vi "N-D TimeStamped Logging (SubVI) v1.0.vi"(8 "error in (no error)":errorcluster, 10 "array":dbl[](array[numeric]), 11 "path":path) -> (0 "error out":errorcluster)   [LabVIEW 2017]
uses:
  <vilib>/Utility/file.llb/Write Delimited Spreadsheet (string).vi
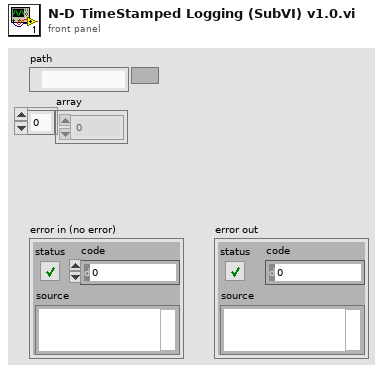
[diagram p1: front panel]
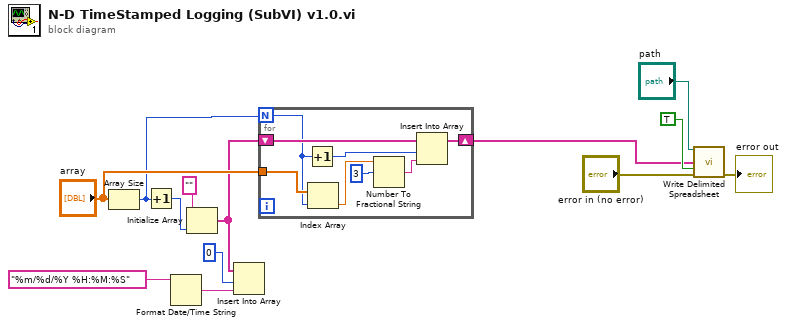
[diagram p0: block diagram]
diagram:
  n1 = Array Size(array="array") -> (size(s)=w6:i32)
  n2 = Increment(x=w6) -> (x+1=w5:i32)
  n3 = Format Date/Time String(time format string (%c)="%m/%d/%Y %H:%M:%S") -> (date/time string=w2:string)  [unwired: 2 in]
  n4 = Initialize Array("" ("element"), w5) -> (w4:string[])
  n5 = Insert Into Array(array=w4, index=0, new element=w2) -> ()  [unwired: 1 out]
  n6 = for {
    N: w6 -> [w15]
    tunnel: "array" -> [w21]
    shift-right: [w16] -> w1
    shift-left: w4 -> [w17]
    n7 = Increment(x=w15) -> (x+1=w14:i32)
    n8 = Index Array(array=w21, index=w15) -> (element=w19:dbl)
    n9 = Number To Fractional String(number=w19, width (-)=i16 3) -> (F-format string=w18:string)  [unwired: 2 in]
    n10 = Insert Into Array(array=w17, index=w14, new element=w18) -> (w16:string[])
  }
  n11 = call-poly <vilib>:"Write Delimited Spreadsheet.vi"("file path (dialog if empty)"="path", "1D data"=w1, "append to file? (new file:F)"=TRUE, "error in (no error)"="error in (no error)") -> ("error out"=→"error out":errorcluster)  [unwired: 10 in, 1 out]
